vi "TrackingAcquisitionLoop.vi"(7 "Image Notifier":refnum<notifier>, 8 "error in (no error)":errorcluster, 9 "Output Data Queue":refnum<queue>, 10 "Input Data Queue":refnum<queue>, 11 "Tracking State Queue":refnum<queue>) -> (0 "error out":errorcluster, 1 "Output Data Queue 2":refnum<queue>, 2 "Input Data Queue 2":refnum<queue>, 5 "Image Notifier Out":refnum<notifier>)   [LabVIEW 2017, in "ImageAcquisitionLibrary.lvlib"]
uses:
  ImageAcquisitionLibrary.lvlib
  Tracking State.ctl
  Acquisition/AcquireData.ctl
  Settings/Settings.ctl
  <vilib>/userdefined/High Color/IMAQdx.ctl
  TrackingSettings.ctl
  Settings/Calibration.ctl
  <vilib>/Utility/error.llb/DialogType.ctl
  SettingsGlobal.vi
panel:
  out "Tracking State Queue 2":refnum<queue>
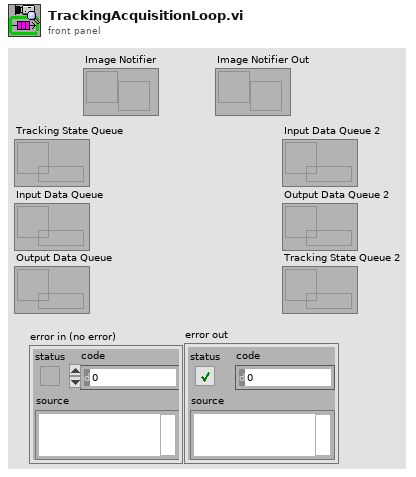
[diagram p1: front panel]
types:
  T1 = typedef "ImageAcquisitionLibrary.lvlib/AcquireData.ctl" = cluster{"Frame Data":cluster{"Image":u32[][], "Timestamp":timestamp, "Image Type":T2, "Dropped Frames":u32}, "Tracking Data":cluster{"Positions":dbl[][], "Timestamp":timestamp}, "Tracked?":bool}
  T2 = typedef "Image Type" = u32
  T3 = typedef "ImageAcquisitionLibrary.lvlib/Settings.ctl" = cluster{"Harware Configuration":cluster{"Camera":T4, "Frames Per Second":u32, "Simulate Recording":bool, "Simulated Recording Sample":path, "Timestamp Method":enum16{"System Timestamp", "Camera Timestamp", "IMAQdx Timestamp"}}, "Base Recording Path":path, "Type Of Recording":string, "Recording Codec":string, "TrackingSettings":T5, "Calibration":T7, "Broadcast Length":i32}
  T4 = typedef "IMAQdx.ctl" = refnum<k21>
  T5 = typedef "ImageAcquisitionLibrary.lvlib/TrackingSettings.ctl" = cluster{"Max Radius":i32, "Threshold":sgl, "ROI":T6}
  T6 = typedef "IMAQ Rectangle" = cluster{"Left":i32, "Top":i32, "Right":i32, "Bottom":i32, "Rotation":dbl}
  T7 = typedef "ImageAcquisitionLibrary.lvlib/Calibration.ctl" = cluster{"Pixel Width (X)":dbl, "Pixel Height (Y)":dbl}
  T8 = typedef "ImageAcquisitionLibrary.lvlib/TrackingImages.ctl" = cluster{"Working Image":T9, "ROI Mask":T9, "Centroid Mask":T9}
  T9 = typedef "IMAQ Image.ctl" = refnum<image>
  T10 = typedef "ImageAcquisitionLibrary.lvlib/Tracking State.ctl" = enum16{"Idle", "Start Tracking", "Track", "Stop Tracking", "Update Settings", "Exit"}
  T11 = typedef "DialogType.ctl" = u16
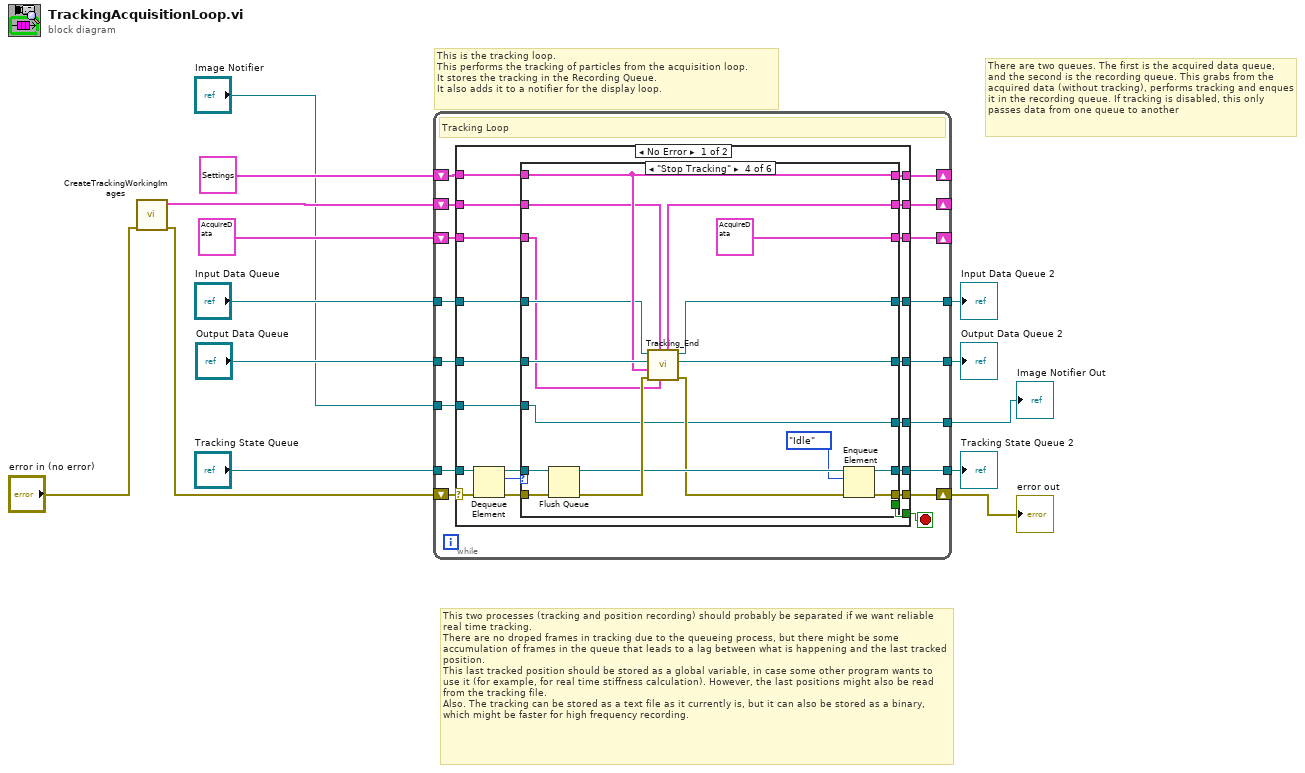
[diagram p0: block diagram]
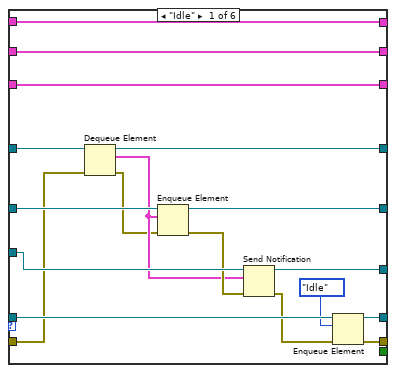
[diagram p2: hidden frame]
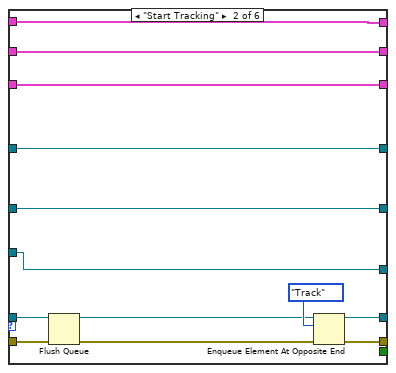
[diagram p3: hidden frame]
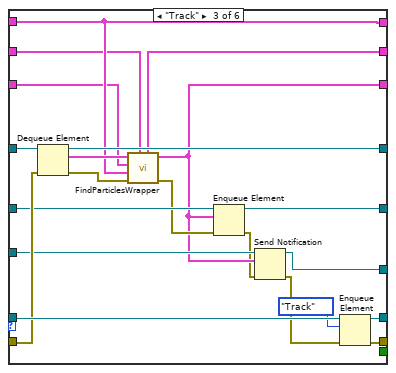
[diagram p4: hidden frame]
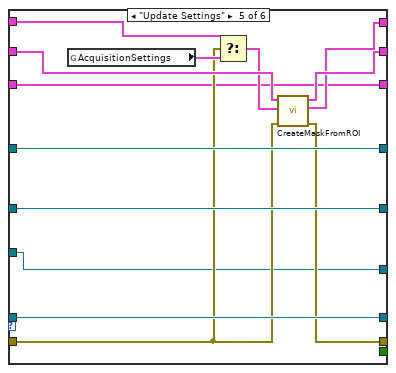
[diagram p5: hidden frame]
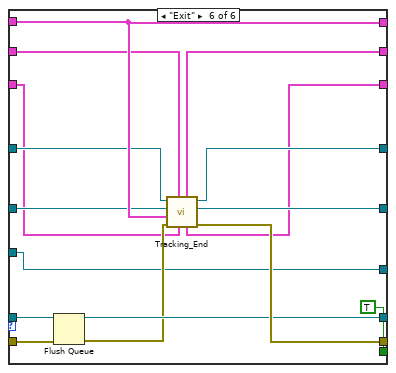
[diagram p6: hidden frame]
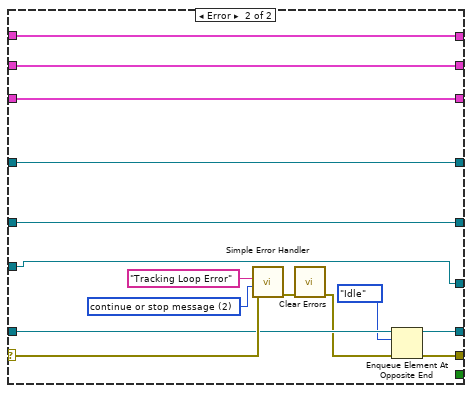
[diagram p7: hidden frame]
diagram:
  # "There are two queues. The first is the acquired data queue, and the second is the recording queue. This grabs from the acquired data (without tracking), performs tracking and enques it in the recording queue. If tracking is disabled, this only passes data from one queue to another"
  # "This two processes (tracking and position recording) should probably be separated if we want reliable real time tracking.\nThere are no droped frames in tracking due to the queueing process, but there might be some accumulation of frames in the queue that leads to a lag between what is happening and the last tracked position. \nThis last tracked position should be stored as a global variable, in case some other program wants to use it (for example, for real time stiffness calculation). However, the last positions might also be read from the tracking file. \nAlso. The tracking can be stored as a text file as it currently is, but it can also be stored as a binary, which might be faster for high frequency recording."
  # "This is the tracking loop.\nThis performs the tracking of particles from the acquisition loop.\nIt stores the tracking in the Recording Queue. \nIt also adds it to a notifier for the display loop."
  n1 = call "CreateTrackingWorkingImages.vi"("error in (no error)"="error in (no error)") -> ("error out"=w3:errorcluster, "Tracking Images"=w4:T8)  [unwired: 9 in]
  n2 = while {
    shift-right: [w24] -> w13
    shift-left: w3 -> [w27]
    shift-right: [w30] -> _
    shift-left: T3 {"Harware Configuration"={"Camera"="cam1", "Frames Per Second"=15, "Simulate Recording"=FALSE, "Simulated Recording Sample"=path "", "Timestamp Method"=enum."Camera Timestamp"}, "Base Recording Path"=path "", "Type Of Recording"="", "Recording Codec"="", "TrackingSettings"={"Max Radius"=0, "Threshold"=160.0, "ROI"={"Left"=0, "Top"=0, "Right"=0, "Bottom"=0, "Rotation"=0.0}}, "Calibration"={"Pixel Width (X)"=10.0, "Pixel Height (Y)"=100.0}, "Broadcast Length"=0} ("Settings") -> [w31]
    tunnel: "Output Data Queue" -> [w29]
    tunnel: "Input Data Queue" -> [w26]
    tunnel: "Tracking State Queue" -> [w25]
    tunnel: [w23] -> w6
    tunnel: [w22] -> w8
    tunnel: [w21] -> w7
    shift-right: [w20] -> _
    shift-left: T1 {"Frame Data"={"Image"=[], "Timestamp"=timestamp(0 s since 1904-01-01), "Image Type"=0, "Dropped Frames"=0}, "Tracking Data"={"Positions"=[], "Timestamp"=timestamp(0 s since 1904-01-01)}, "Tracked?"=FALSE} ("Acquired Data") -> [w19]
    shift-right: [w17] -> _
    shift-left: w4 -> [w18]
    tunnel: "Image Notifier" -> [w16]
    tunnel: [w15] -> w1
    stop <- w28 stop-if-true
    # "Tracking Loop"
    n3 = case shown="No Error" w27 {
      selector: w27 -> [w44 w164]
      tunnel: w31 -> [w51 w165]
      tunnel: [w50 w165] -> w30
      tunnel: w29 -> [w49 w158]
      tunnel: [w48 _] -> w28
      tunnel: w26 -> [w47 w159]
      tunnel: w25 -> [w46 w155]
      tunnel: [w43 w152] -> w24
      tunnel: [w40 w154] -> w23
      tunnel: [w39 w159] -> w22
      tunnel: [w38 w158] -> w21
      tunnel: [w37 w160] -> w20
      tunnel: w19 -> [w34 w160]
      tunnel: w18 -> [w36 w157]
      tunnel: [w35 w157] -> w17
      tunnel: w16 -> [w33 w156]
      tunnel: [w32 w156] -> w15
      frame No Error {
        n4 = Dequeue Element(queue=w46, error in (no error)=w44) -> (queue out=w41:refnum<queue>, element=w45:T10, error out=w42:errorcluster)  [unwired: 1 in, 1 out]
        n5 = case shown="\"Stop Tracking\"" w45 {
          tunnel: w51 -> [w69 w82 w91 w120 w133 w149]
          tunnel: [w69 w82 w91 w120 w124 w149] -> w50
          tunnel: w49 -> [w68 w80 w95 w121 w131 w144]
          tunnel: [_ _ _ _ _ TRUE] -> w48
          tunnel: w47 -> [w56 w81 w99 w118 w132 w145]
          tunnel: [w66 w76 w101 w109 w126 w146] -> w43
          tunnel: w42 -> [w53 w70 w98 w116 w127 w147]
          tunnel: w41 -> [w65 w73 w102 w115 w130 w148]
          tunnel: [w64 w79 w100 w112 w130 w141] -> w40
          tunnel: [w55 w81 w97 w113 w132 w142] -> w39
          tunnel: [w67 w80 w93 w114 w131 w143] -> w38
          tunnel: [w61 w75 w86 T1 {"Frame Data"={"Image"=[], "Timestamp"=timestamp(0 s since 1904-01-01), "Image Type"=0, "Dropped Frames"=0}, "Tracking Data"={"Positions"=[], "Timestamp"=timestamp(0 s since 1904-01-01)}, "Tracked?"=FALSE} ("Data Out") w123 w137] -> w37
          tunnel: w36 -> [w62 w77 w90 w106 w129 w139]
          tunnel: [w62 w77 w89 w105 w128 w138] -> w35
          tunnel: w34 -> [w61 w75 w88 w107 w123 w136]
          tunnel: w33 -> [w60 w74 w87 w104 w122 w135]
          tunnel: [w57 w74 w83 w104 w122 w135] -> w32
          frame "Idle" {
            n6 = Dequeue Element(queue=w56, error in (no error)=w53) -> (queue out=w55:refnum<queue>, element=w54:T1, error out=w52:errorcluster)  [unwired: 1 in, 1 out]
            n7 = Enqueue Element(queue=w68, element=w54, error in (no error)=w52) -> (queue out=w67:refnum<queue>, error out=w59:errorcluster)  [unwired: 1 in, 1 out]
            n8 = Send Notification(notification=w54, notifier=w60, error in (no error)=w59) -> (notifier out=w57:refnum<notifier>, error out=w58:errorcluster)
            n9 = Enqueue Element(queue=w65, element=Tracking_State."Idle", error in (no error)=w58) -> (queue out=w64:refnum<queue>, error out=w66:errorcluster)  [unwired: 1 in, 1 out]
          }
          frame "Start Tracking" {
            n10 = Flush Queue(queue=w73, error in (no error)=w70) -> (queue out=w72:refnum<queue>, error out=w71:errorcluster)  [unwired: 1 out]
            n11 = Enqueue Element At Opposite End(queue=w72, element=Tracking_State."Track", error in (no error)=w71) -> (queue out=w79:refnum<queue>, error out=w76:errorcluster)  [unwired: 1 in, 1 out]
          }
          frame "Track" {
            n12 = Dequeue Element(queue=w99, error in (no error)=w98) -> (queue out=w97:refnum<queue>, element=w96:T1, error out=w103:errorcluster)  [unwired: 1 in, 1 out]
            n13 = call "FindParticlesWrapper.vi"(7:w90, "error in"=w103, "Settings"=w91, "Data Old"=w88, "Data"=w96) -> ("error out"=w94:errorcluster, "Data Out"=w86:T1, 5:w89:T8)  [unwired: 4 in]
            n14 = Enqueue Element(queue=w95, element=w86, error in (no error)=w94) -> (queue out=w93:refnum<queue>, error out=w85:errorcluster)  [unwired: 1 in, 1 out]
            n15 = Send Notification(notification=w86, notifier=w87, error in (no error)=w85) -> (notifier out=w83:refnum<notifier>, error out=w84:errorcluster)
            n16 = Enqueue Element(queue=w102, element=Tracking_State."Track", error in (no error)=w84) -> (queue out=w100:refnum<queue>, error out=w101:errorcluster)  [unwired: 1 in, 1 out]
          }
          frame "Stop Tracking" {
            n17 = Flush Queue(queue=w115, error in (no error)=w116) -> (queue out=w111:refnum<queue>, error out=w119:errorcluster)  [unwired: 1 out]
            n18 = call "Tracking_End.vi"("Last Frame Data"=w107, 7:w106, "error in"=w119, "Settings"=w120, "Output Data Queue"=w121, "Input Data Queue"=w118) -> ("error out"=w110:errorcluster, "Output Data Queue"=w114:refnum<queue>, "Input Data Queue 2"=w113:refnum<queue>, 5:w105:T8)  [unwired: 1 in, 1 out]
            n19 = Enqueue Element(queue=w111, element=Tracking_State."Idle", error in (no error)=w110) -> (queue out=w112:refnum<queue>, error out=w109:errorcluster)  [unwired: 1 in, 1 out]
          }
          frame "Update Settings" {
            n20 = global read "SettingsGlobal.vi" "AcquisitionSettings"() -> (w134:T3)
            n21 = Select(t=w133, s=w127, f=w134) -> (s? t:f=w125:T3)
            n22 = call "CreateMaskFromROI.vi"("error in (no error)"=w127, "Settings"=w125, 11:w129) -> ("error out"=w126:errorcluster, "Settings 2"=w124:T3, "output cluster"=w128:T8)  [unwired: 6 in]
          }
          frame "Exit" {
            n23 = Flush Queue(queue=w148, error in (no error)=w147) -> (queue out=w141:refnum<queue>, error out=w140:errorcluster)  [unwired: 1 out]
            n24 = call "Tracking_End.vi"("Last Frame Data"=w136, 7:w139, "error in"=w140, "Settings"=w149, "Output Data Queue"=w144, "Input Data Queue"=w145) -> ("error out"=w146:errorcluster, "Output Data Queue"=w143:refnum<queue>, "Input Data Queue 2"=w142:refnum<queue>, "Last Frame Data Out"=w137:T1, 5:w138:T8)  [unwired: 1 in]
          }
        }
      }
      frame Error {
        w163 = T11 2 items=["no dialog", "OK message", "continue or stop message", "OK message + warnings", "continue/stop + warnings"] ("type of dialog (OK msg:1)")
        n25 = call <vilib>:"Simple Error Handler.vi"("error source (\" \")"="Tracking Loop Error" ("error source (\" \")"), "type of dialog (OK msg:1)"=w163, "error in (no error)"=w164) -> ("error out"=w162:errorcluster)  [unwired: 2 in, 4 out]
        n26 = call <vilib>:"Clear Errors.vi"("error in (no error)"=w162) -> ("error out"=w153:errorcluster)  [unwired: 5 in, 1 out]
        n27 = Enqueue Element At Opposite End(queue=w155, element=Tracking_State."Idle", error in (no error)=w153) -> (queue out=w154:refnum<queue>, error out=w152:errorcluster)  [unwired: 1 in, 1 out]
      }
    }
  }
  "error out" <- w13
  "Input Data Queue 2" <- w8
  "Output Data Queue 2" <- w7
  "Tracking State Queue 2" <- w6
  "Image Notifier Out" <- w1
